vi "Registry.vi"(3 "OpenedVI":cluster{"ViReference":refnum<vi>, "Path":string}, 4 "Client":cluster{"Address":string, "Port":u16}, 5 "ParserReferecne":refnum<vi>, 6 "Command":T2(ring)) -> (0 "RegText":string, 1 "ConectionsNumber":i32, 2 "VI_in_use?":bool)   [LabVIEW 2010]
uses:
  GlobalRegistry.vi
panel:
  out "Temp":T1(array[cluster])
  out "error out":errorcluster
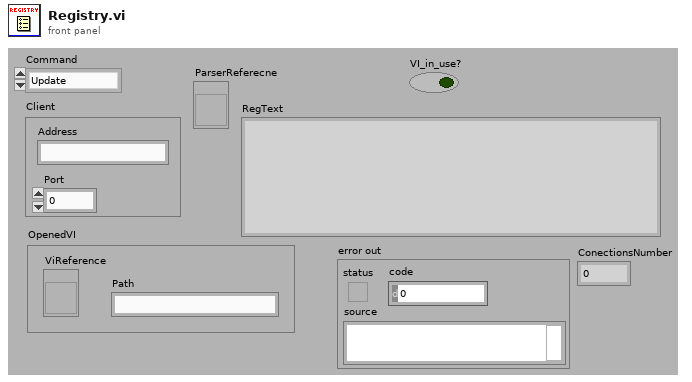
[diagram p1: front panel]
types:
  T1 = cluster{"Pharser reference":refnum<vi>, "remote address":string, "remote port":u16, "path":string, "VI reference":refnum<vi>}[]
  T2 = enum16{"Update", "registry", "Init", "clean", "Close"}
  T3 = enum32{"Bad", "Idle", "Run top level", "Running"}
  T4 = cluster{"Pharser reference":refnum<vi>, "remote address":string, "remote port":u16, "path":string, "VI reference":refnum<vi>}
  T5 = cluster{"ParserReferecne":refnum<vi>, "Address":string, "Port":u16, string, "ViReference 2":refnum<vi>}
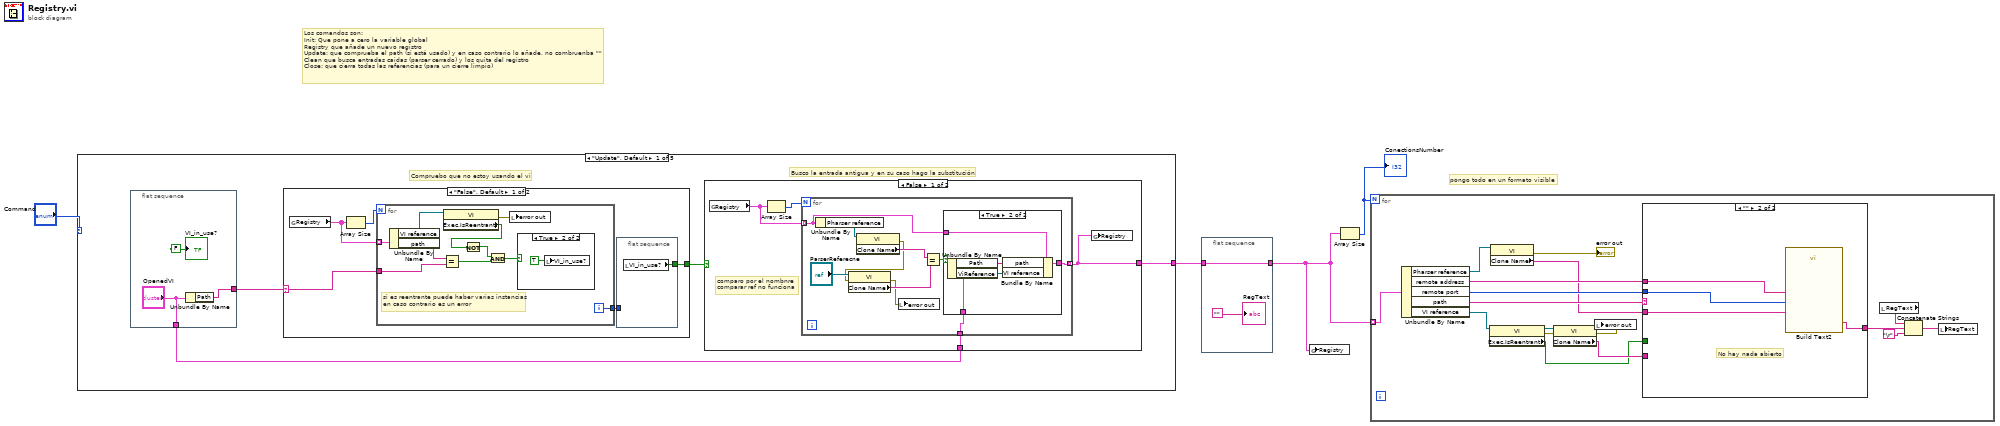
[diagram p0: block diagram]
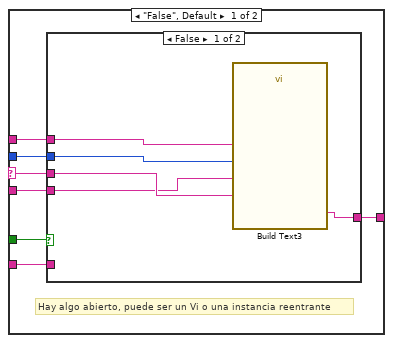
[diagram p2: hidden frame]
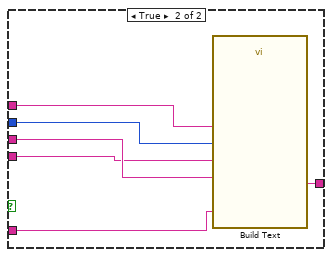
[diagram p3: hidden frame]
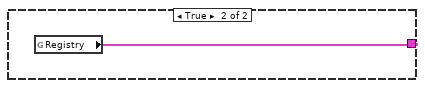
[diagram p5: hidden frame]
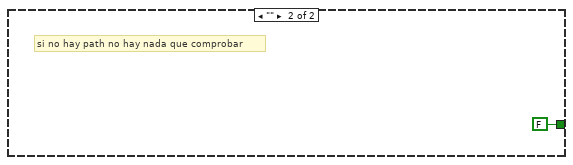
[diagram p7: hidden frame]
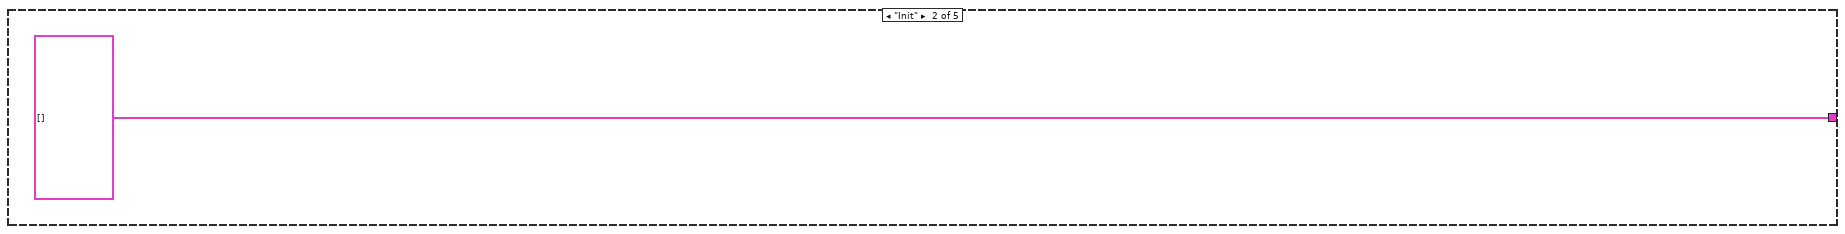
[diagram p8: hidden frame]
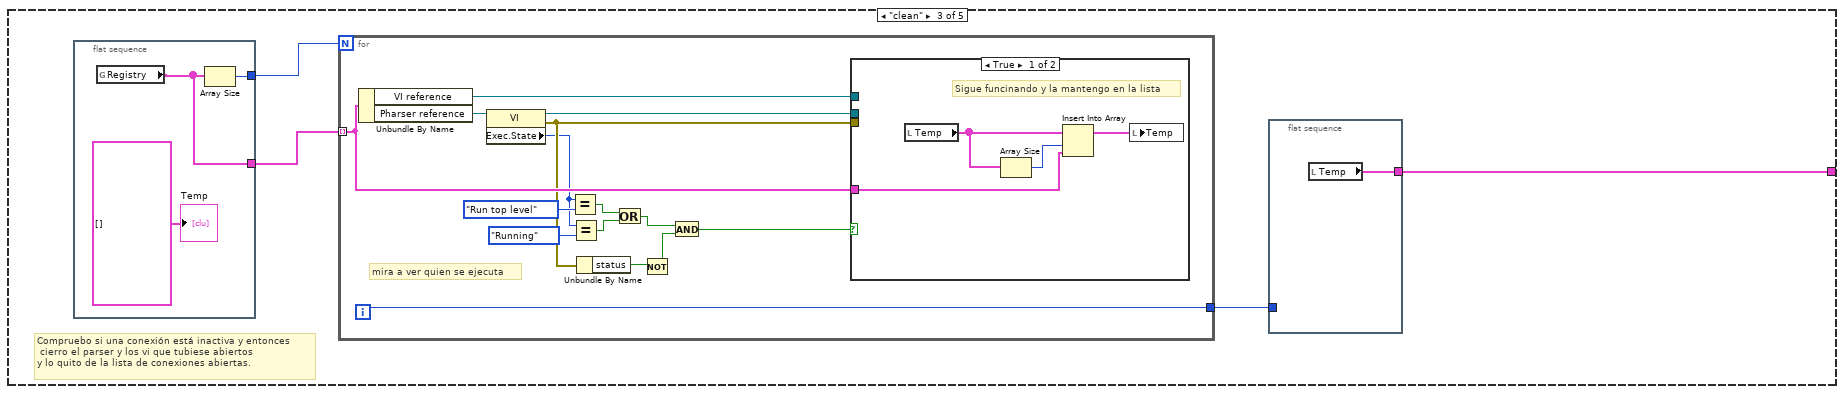
[diagram p9: hidden frame]
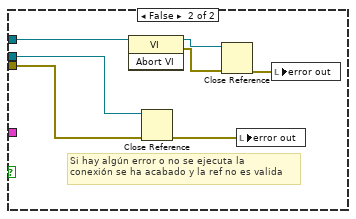
[diagram p10: hidden frame]
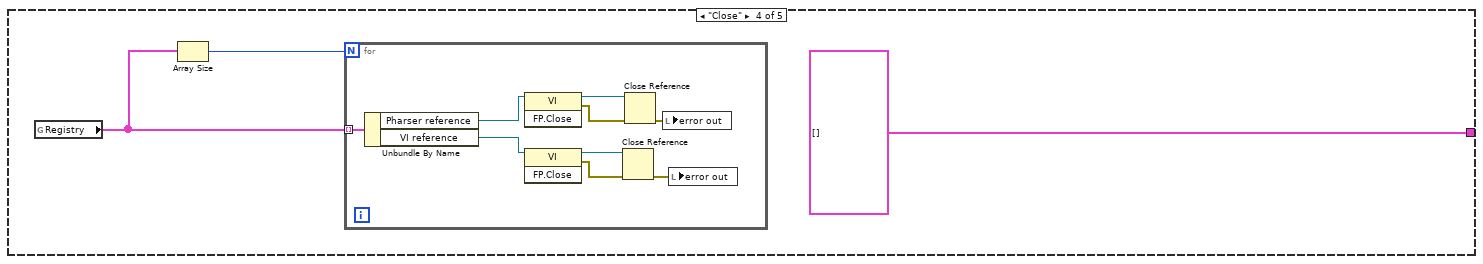
[diagram p11: hidden frame]
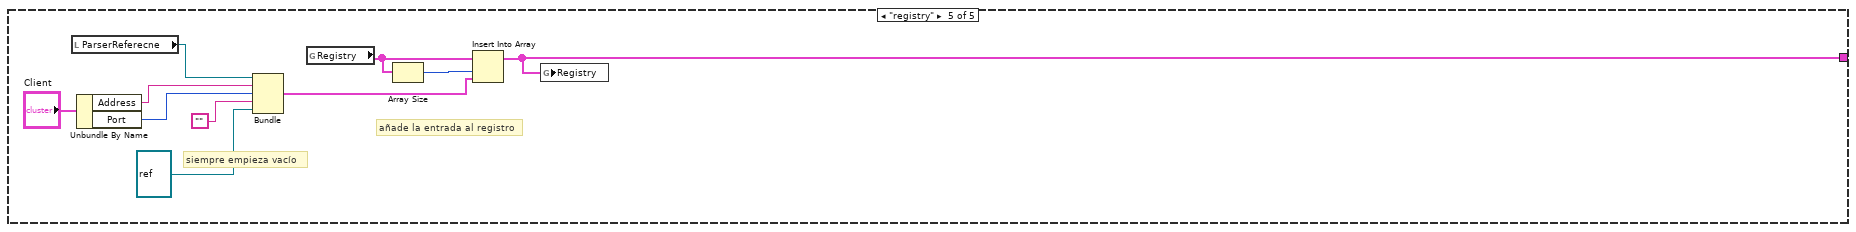
[diagram p12: hidden frame]
diagram:
  # "pongo todo en un formato visible"
  # "Los comandos son:\nInit: Que pone a cero la variable global\nRegistry que añade un nuevo registro\nUpdate: que comprueba el path (si está usado) y en caso contrario lo añade, no combruenba \"\"\nClean que busca entradas caidas (parser cerrado) y los quita del registro\nClose: que cierra todas las referencias (para un cierre limpio)"
  n1 = case shown="\"Update\", Default" "Command" {
    tunnel: [w8 T1 [] ("Registry") w52 T1 [] ("Registry") w102] -> w2
    frame "Update", Default {
      # "Busco la entrada antigua y en su caso hago la substitución"
      # "Compruebo que no estoy usando el vi"
      n2 = flat-sequence {
        tunnel: [w31] -> w5
        tunnel: ["OpenedVI"] -> w6
        frame #0 {
          n3 = Unbundle By Name("OpenedVI") -> ("Path"=w31:string)
          "VI_in_use?" <- FALSE
        }
      }
      n4 = case shown="\"False\", Default" w5 {
        selector: w5 -> [w35 _]
        tunnel: [w34 FALSE ("VI_in_use?")] -> w7
        frame "False", Default {
          n5 = global read "GlobalRegistry.vi" "Registry"() -> (w36:T1)
          n6 = Array Size(array=w36) -> (size(s)=w37:i32)
          n7 = for {
            N: w37 -> [_]
            tunnel: w36 -> [w48] mode=indexing
            tunnel: w35 -> [w46]
            tunnel: [w45] -> w33
            i -> [w45]
            # "si es reentrante puede haber varias instancias\nen caso contrario es un error"
            n8 = Unbundle By Name(w48) -> ("VI reference"=w44:refnum<vi>, "path"=w47:string)
            n9 = Equal?(x=w47, y=w46) -> (x = y?=w39:bool)
            n10 = property class="VI"(reference=w44) -> (error out=w43:errorcluster, "Exec.IsReentrant"=w42:bool)  [unwired: 1 in, 1 out]
            n11 = Not(x=w42) -> (.not. x?=w40:bool)
            n12 = And(x=w40, y=w39) -> (x .and. y?=w41:bool)
            n13 = local write "error out"(w43) -> ()
            n14 = case shown="True" w41 {
              frame False {
              }
              frame True {
                n15 = local write "VI_in_use?"(TRUE ("VI_in_use?")) -> ()
              }
            }
          }
          n16 = flat-sequence {
            tunnel: [w38] -> w34
            tunnel: w33 -> [_]
            frame #0 {
              n17 = local read "VI_in_use?"() -> (w38:bool)
            }
          }
        }
        frame "" {
          # "si no hay path no hay nada que comprobar"
        }
      }
      n18 = case shown="False" w7 {
        tunnel: [w9 w29] -> w8
        tunnel: w6 -> [w10 _]
        frame False {
          # "comparo por el nombnre\ncomparar ref no funciona"
          n19 = global read "GlobalRegistry.vi" "Registry"() -> (w11:T1)
          n20 = Array Size(array=w11) -> (size(s)=w12:i32)
          n21 = for {
            N: w12 -> [_]
            tunnel: w11 -> [w21] mode=indexing
            tunnel: w10 -> [w20]
            tunnel: [w19] -> w9 mode=indexing
            n22 = Unbundle By Name(w21) -> ("Pharser reference"=w18:refnum<vi>)
            n23 = property class="VI"(reference=w18) -> (error out=w14:errorcluster, "Clone Name"=w16:string)  [unwired: 1 in, 1 out]
            n24 = property class="VI"(reference="ParserReferecne", error in=w14) -> (error out=w13:errorcluster, "Clone Name"=w15:string)  [unwired: 1 out]
            n25 = local write "error out"(w13) -> ()
            n26 = Equal?(x=w16, y=w15) -> (x = y?=w22:bool)
            n27 = case shown="True" w22 {
              tunnel: w21 -> [w23 w28]
              tunnel: w20 -> [_ w26]
              tunnel: [w23 w27] -> w19
              frame False {
              }
              frame True {
                n28 = Unbundle By Name(w26) -> ("Path"=w24:string, "ViReference"=w25:refnum<vi>)
                n29 = Bundle By Name(cluster=w28, "path"=w24, "VI reference"=w25) -> (w27:T4)
              }
            }
          }
          n30 = global write "GlobalRegistry.vi" "Registry"(w9) -> ()
        }
        frame True {
          n31 = global read "GlobalRegistry.vi" "Registry"() -> (w29:T1)
        }
      }
    }
    frame "Init" {
    }
    frame "clean" {
      # "Compruebo si una conexión está inactiva y entonces\n cierro el parser y los vi que tubiese abiertos\ny lo quito de la lista de conexiones abiertas."
      n32 = flat-sequence {
        tunnel: [w59] -> w55
        tunnel: [w58] -> w54
        frame #0 {
          n33 = global read "GlobalRegistry.vi" "Registry"() -> (w58:T1)
          n34 = Array Size(array=w58) -> (size(s)=w59:i32)
          "Temp" <- T1 [] ("Temp")
        }
      }
      n35 = for {
        N: w55 -> [_]
        tunnel: w54 -> [w72] mode=indexing
        tunnel: [w71] -> w53
        i -> [w71]
        # "mira a ver quien se ejecuta"
        n36 = Unbundle By Name(w72) -> ("VI reference"=w60:refnum<vi>, "Pharser reference"=w74:refnum<vi>)
        n37 = property class="VI"(reference=w74) -> (reference out=w73:refnum<vi>, error out=w68:errorcluster, "Exec.State"=w62:T3)  [unwired: 1 in]
        n38 = Equal?(x=w62, y=T3."Run top level") -> (x = y?=w64:bool)
        n39 = Equal?(x=w62, y=T3."Running") -> (x = y?=w63:bool)
        n40 = Unbundle By Name(w68) -> ("status"=w67:bool)
        n41 = Or(x=w64, y=w63) -> (x .or. y?=w65:bool)
        n42 = Not(x=w67) -> (.not. x?=w66:bool)
        n43 = And(x=w65, y=w66) -> (x .and. y?=w61:bool)
        n44 = case shown="True" w61 {
          tunnel: w73 -> [_ w83]
          tunnel: w72 -> [w75 _]
          tunnel: w68 -> [_ w85]
          tunnel: w60 -> [_ w82]
          frame True {
            # "Sigue funcinando y la mantengo en la lista"
            n45 = local read "Temp"() -> (w78:T1)
            n46 = Array Size(array=w78) -> (size(s)=w77:i32)
            n47 = Insert Into Array(array=w78, index=w77, new element=w75) -> (w76:T1)
            n48 = local write "Temp"(w76) -> ()
          }
          frame False {
            # "Si hay algún error o no se ejecuta la\nconexión se ha acabado y la ref no es valida"
            n49 = invoke class="VI" method="Abort VI"(reference=w82) -> (reference out=w81:refnum<vi>, error out=w80:errorcluster)  [unwired: 2 in, 1 out]
            n50 = Close Reference(reference=w83, error in (no error)=w85) -> (error out=w84:errorcluster)
            n51 = Close Reference(reference=w81, error in (no error)=w80) -> (error out=w79:errorcluster)
            n52 = local write "error out"(w84) -> ()
            n53 = local write "error out"(w79) -> ()
          }
        }
      }
      n54 = flat-sequence {
        tunnel: w53 -> [_]
        tunnel: [w56] -> w52
        frame #0 {
          n55 = local read "Temp"() -> (w56:T1)
        }
      }
    }
    frame "Close" {
      n56 = global read "GlobalRegistry.vi" "Registry"() -> (w87:T1)
      n57 = Array Size(array=w87) -> (size(s)=w88:i32)
      n58 = for {
        N: w88 -> [_]
        tunnel: w87 -> [w97] mode=indexing
        n59 = Unbundle By Name(w97) -> ("Pharser reference"=w90:refnum<vi>, "VI reference"=w89:refnum<vi>)
        n60 = invoke class="VI" method="FP.Close"(reference=w90) -> (reference out=w91:refnum<vi>, error out=w92:errorcluster)  [unwired: 2 in, 1 out]
        n61 = invoke class="VI" method="FP.Close"(reference=w89) -> (reference out=w93:refnum<vi>, error out=w94:errorcluster)  [unwired: 2 in, 1 out]
        n62 = Close Reference(reference=w93, error in (no error)=w94) -> (error out=w96:errorcluster)
        n63 = Close Reference(reference=w91, error in (no error)=w92) -> (error out=w95:errorcluster)
        n64 = local write "error out"(w95) -> ()
        n65 = local write "error out"(w96) -> ()
      }
    }
    frame "registry" {
      # "siempre empieza vacío"
      # "añade la entrada al registro"
      n66 = local read "ParserReferecne"() -> (w105:refnum<vi>)
      n67 = Unbundle By Name("Client") -> ("Address"=w99:string, "Port"=w100:u16)
      n68 = Bundle("ParserReferecne"=w105, "Address"=w99, "Port"=w100, "", "ViReference 2"=refnum<vi> refnum) -> (w103:T5)  [unwired: 1 in]
      n69 = global read "GlobalRegistry.vi" "Registry"() -> (w106:T1)
      n70 = Array Size(array=w106) -> (size(s)=w107:i32)
      n71 = Insert Into Array(array=w106, index=w107, new element=w103) -> (w102:T1)
      n72 = global write "GlobalRegistry.vi" "Registry"(w102) -> ()
    }
  }
  n73 = flat-sequence {
    tunnel: [w108] -> w1
    tunnel: w2 -> [w108]
    frame #0 {
      "RegText" <- ""
    }
  }
  n74 = global write "GlobalRegistry.vi" "Registry"(w1) -> ()
  n75 = Array Size(array=w1) -> (size(s)=w3:i32)
  "ConectionsNumber" <- w3
  n76 = for {
    N: w3 -> [_]
    tunnel: w1 -> [w126] mode=indexing
    n77 = Unbundle By Name(w126) -> ("Pharser reference"=w118:refnum<vi>, "remote address"=w124:string, "remote port"=w123:u16, "path"=w125:string, "VI reference"=w115:refnum<vi>)
    n78 = property class="VI"(reference=w115) -> (reference out=w114:refnum<vi>, error out=w111:errorcluster, "Exec.IsReentrant"=w110:bool)  [unwired: 1 in]
    n79 = property class="VI"(reference=w118) -> (error out=→"error out":errorcluster, "Clone Name"=w116:string)  [unwired: 1 in, 1 out]
    n80 = property class="VI"(reference=w114, error in=w111) -> (error out=w112:errorcluster, "Clone Name"=w113:string)  [unwired: 1 out]
    n81 = local write "error out"(w112) -> ()
    n82 = case shown="\"\"" w125 {
      selector: w125 -> [w131 _]
      tunnel: w124 -> [w133 w148]
      tunnel: w123 -> [w132 w147]
      tunnel: [w130 w146] -> w119
      tunnel: w116 -> [w129 w145]
      tunnel: w110 -> [w128 _]
      tunnel: w113 -> [w127 _]
      frame "False", Default {
        # "Hay algo abierto, puede ser un Vi o una instancia reentrante"
        n83 = case shown="False" w128 {
          tunnel: w133 -> [w138 w144]
          tunnel: w132 -> [w137 w143]
          tunnel: w131 -> [w136 w142]
          tunnel: [w134 w141] -> w130
          tunnel: w129 -> [w135 w140]
          tunnel: w127 -> [_ w139]
          frame False {
            n84 = call "Build Text3"("path"=w136, "IP"=w138, "port"=w137, "parser"=w135) -> ("Result"=w134:string)  [unwired: 10 in, 1 out]
          }
          frame True {
            n85 = call "Build Text"("path"=w142, "IP"=w144, "port"=w143, "parser"=w140, "name"=w139) -> ("Result"=w141:string)  [unwired: 9 in, 1 out]
          }
        }
      }
      frame "" {
        # "No hay nada abierto"
        n86 = call "Build Text2"("IP"=w148, "port"=w147, "parser"=w145) -> ("Result"=w146:string)  [unwired: 11 in, 1 out]
      }
    }
    n87 = local read "RegText"() -> (w122:string)
    n88 = Concatenate Strings(w122, w119, "\r") -> (w121:string)
    n89 = local write "RegText"(w121) -> ()
  }
